vi "LAB6.vi"() -> ()   [LabVIEW 2023]
panel:
  out "Rang":u8
  out "Minimul de rang par":dbl
  out "Rang":u8
  out "Maxim de rang impar":dbl
  out "Sir monoton":bool
  out "Valori intre a si b":dbl[](array[numeric])
  in  "b":dbl
  in  "a":dbl
  in  "Array initial":dbl[](array[numeric])
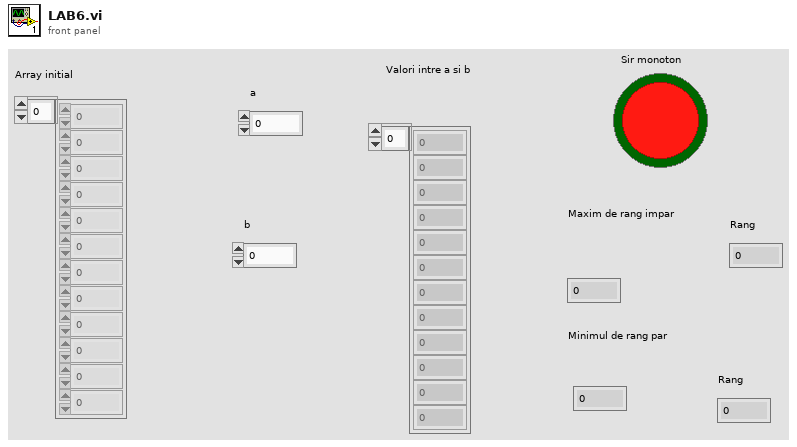
[diagram p1: front panel]
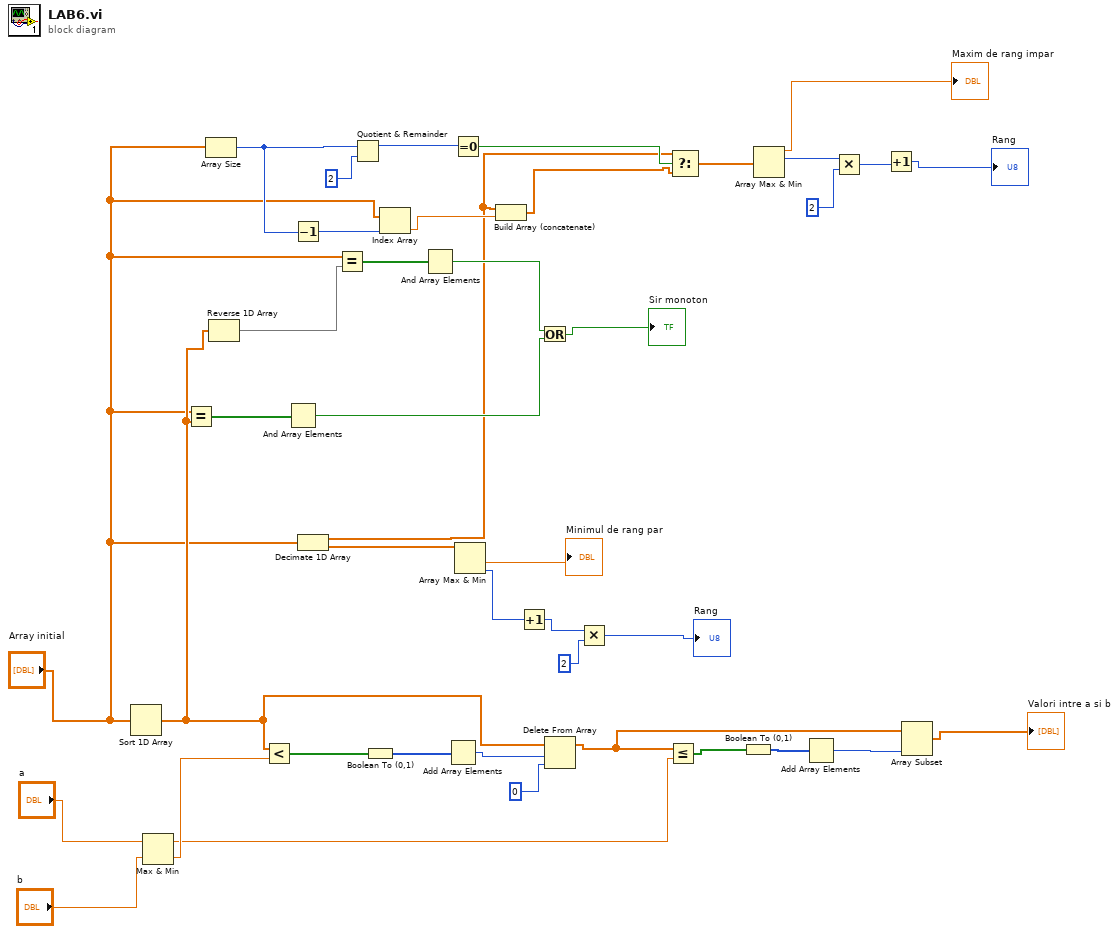
[diagram p0: block diagram]
diagram:
  n1 = Sort 1D Array(array="Array initial") -> (sorted array=w27:dbl[])
  n2 = Max & Min(x="a", y="b") -> (max(x,y)=w34:dbl, min(x,y)=w39:dbl)
  n3 = Equal?(x="Array initial", y=w27) -> (x = y?=w28:bool[])
  n4 = Array Size(array="Array initial") -> (size(s)=w14:i32)
  n5 = Reverse 1D Array(array=w27) -> (reversed array=w26:dbl[])
  n6 = Less?(x=w27, y=w39) -> (x < y?=w38:bool[])
  n7 = And Array Elements(Boolean array=w28) -> (logical AND=w24:bool)
  n8 = Decrement(x=w14) -> (x-1=w13:i32)
  n9 = Decimate 1D Array "Decimate 1D Array"("Array initial") -> (w1:dbl[], w9:dbl[])
  n10 = Equal?(x="Array initial", y=w26) -> (x = y?=w25:bool[])
  n11 = Quotient & Remainder(x=w14, y=2) -> (x-y*floor(x/y)=w15:i32)  [unwired: 1 out]
  n12 = Boolean To (0,1)(Boolean=w38) -> (0, 1=w37:i16[])
  n13 = Index Array "Index Array"(array="Array initial", index=w13) -> (element=w11:dbl)
  n14 = And Array Elements(Boolean array=w25) -> (logical AND=w23:bool)
  n15 = Add Array Elements(numeric array=w37) -> (sum=w36:i16)
  n16 = Equal To 0?(x=w15) -> (x = 0?=w10:bool)
  n17 = Array Max & Min(array=w9) -> (min value=→"Minimul de rang par":dbl, min index (indices)=w20:i32)  [unwired: 2 out]
  n18 = Build Array (concatenate) "Build Array"(w1, w11) -> (w8:dbl[])
  n19 = Increment(x=w20) -> (x+1=w19:i32)
  n20 = Or(x=w23, y=w24) -> (x .or. y?=→"Sir monoton":bool)
  n21 = Delete From Array(array=w27, length=w36, index=0) -> (array with subset deleted=w30:dbl[])  [unwired: 1 out]
  n22 = Multiply(x=w19, y=2) -> (x*y=→"Rang":i32)
  n23 = Less Or Equal?(x=w30, y=w34) -> (x <= y?=w33:bool[])
  n24 = Select(t=w1, s=w10, f=w8) -> (s? t:f=w7:dbl[])
  n25 = Boolean To (0,1)(Boolean=w33) -> (0, 1=w32:i16[])
  n26 = Array Max & Min(array=w7) -> (max value=→"Maxim de rang impar":dbl, max index (indices)=w6:i32)  [unwired: 2 out]
  n27 = Add Array Elements(numeric array=w32) -> (sum=w31:i16)
  n28 = Multiply(x=w6, y=2) -> (x*y=w4:i32)
  n29 = Increment(x=w4) -> (x+1=→"Rang":i32)
  n30 = Array Subset(array=w30, length=w31) -> (→"Valori intre a si b":dbl[])  [unwired: 1 in]
